vi "IRISS V2 Get Joint Cmd.vi"(5 "Left or Right Arm":i32(ring)=1 items=["Left Arm", "Right Arm"]) -> (1 "Joint Cmd Posit":dbl[](array[numeric]))   [LabVIEW 2016]
uses:
  EyeRobotDLL.dll
panel:
  out "grasp":dbl
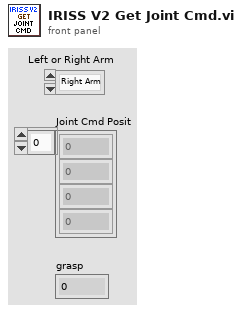
[diagram p1: front panel]
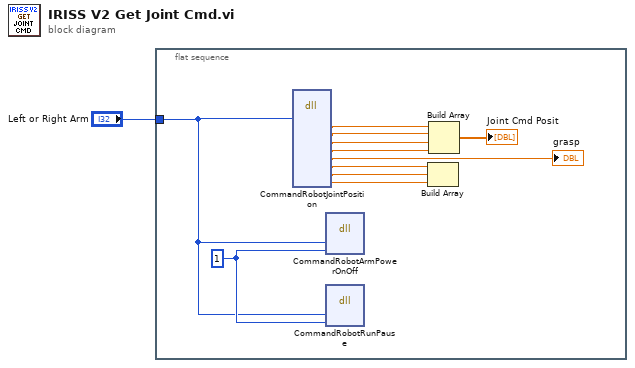
[diagram p0: block diagram]
diagram:
  n1 = flat-sequence {
    tunnel: "Left or Right Arm" -> [w10]
    frame #0 {
      w12 = 1 ("OnOff")
      n2 = dll-call lib="D:/IRISSoft LV2016 beta/Host Demo/Functions/EyeRobotDLL.dll" fn="CommandRobotJointPosition"("id"=w10) -> ("j0"=w9:dbl, "j1"=w8:dbl, "j2"=w7:dbl, "j3"=w6:dbl, "j4"=→"grasp":dbl, "j5"=w4:dbl, "j6"=w3:dbl, "j7"=w2:dbl)  [unwired: 13 in, 2 out]
      n3 = dll-call lib="D:/IRISSoft LV2016 beta/Host Demo/Functions/EyeRobotDLL.dll" fn="CommandRobotArmPowerOnOff"("id"=w10, "OnOff"=w12) -> ()  [unwired: 6 in, 2 out]
      n4 = dll-call lib="D:/IRISSoft LV2016 beta/Host Demo/Functions/EyeRobotDLL.dll" fn="CommandRobotRunPause"("id"=w10, "RunPause"=w12) -> ()  [unwired: 6 in, 2 out]
      n5 = Build Array(w4, w3, w2) -> ()  [unwired: 1 out]
      n6 = Build Array(w9, w8, w7, w6) -> (→"Joint Cmd Posit":dbl[])
    }
  }
